vi "BallShear_BallSelection.vi"(8 "Selected Balls":dbl[][](array[numeric]), 11 "Check":bool) -> (3 "Ready":bool)   [LabVIEW 2013]
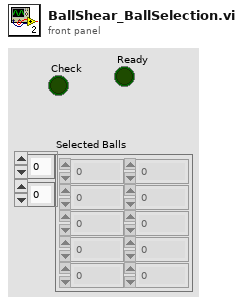
[diagram p1: front panel]
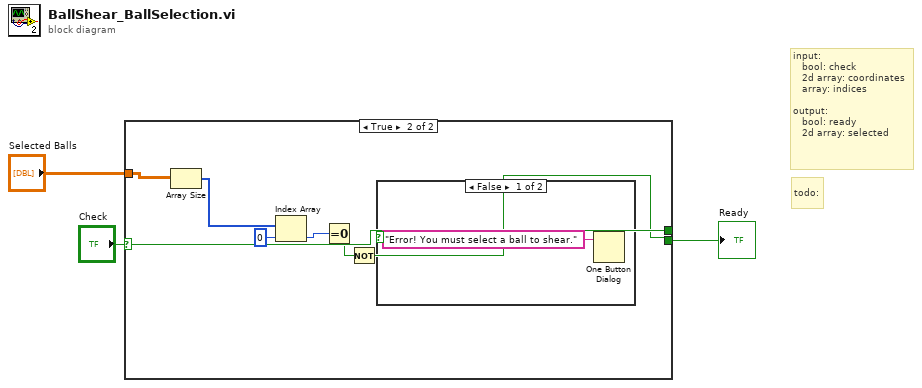
[diagram p0: block diagram]
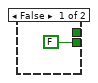
[diagram p2: hidden frame]
diagram:
  # "input:\n   bool: check\n   2d array: coordinates\n   array: indices\n\noutput: \n   bool: ready\n   2d array: selected"
  # "todo:"
  n1 = case shown="True" "Check" {
    tunnel: "Check" -> [_ _]
    tunnel: [FALSE ("Power") w5] -> w2
    tunnel: "Selected Balls" -> [_ w10]
    frame False {
    }
    frame True {
      n2 = Array Size(array=w10) -> (size(s)=w9:i32[])
      n3 = Index Array(array=w9, index=0) -> (element=w7:i32)
      n4 = Equal To 0?(x=w7) -> (x = 0?=w6:bool)
      n5 = Not(x=w6) -> (.not. x?=w5:bool)
      n6 = case shown="False" w5 {
        frame False {
          n7 = One Button Dialog(message="Error! You must select a ball to shear.") -> ()  [unwired: 1 in, 1 out]
        }
        frame True {
        }
      }
    }
  }
  "Ready" <- w2
